vi "Generate stitch tier template.vi"(8 "error in (no error)":errorcluster, 10 "Which tier?":enum16{"Top tier", "Bottom tier"}(ring), 11 "Input image":T1) -> (0 "error out":errorcluster, 3 "Tier image template":T1)   [LabVIEW 2020]
uses:
  <vilib>/vision/Image Controls.llb/IMAQ Image.ctl
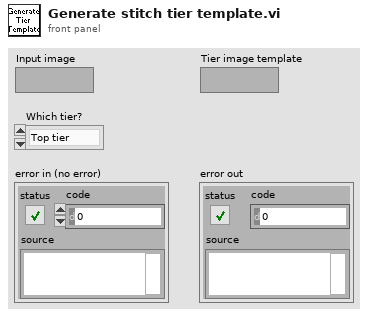
[diagram p1: front panel]
types:
  T1 = typedef "IMAQ Image.ctl" = refnum<image>
  T2 = typedef "Image Type" = u32
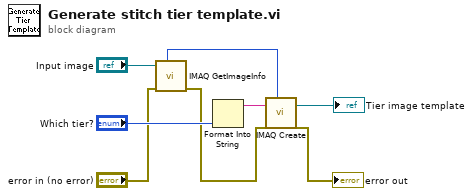
[diagram p0: block diagram]
diagram:
  n1 = call "IMAQ GetImageInfo"("error in (no error)"="error in (no error)", "Image"="Input image") -> ("error out"=w2:errorcluster, "Image Type"=w8:T2)  [unwired: 2 in, 6 out]
  n2 = Format Into String("Which tier?") -> (resulting string=w6:string)  [unwired: 3 in, 1 out]
  n3 = call "IMAQ Create"("Image Name"=w6, "Image Type"=w8, "error in (no error)"=w2) -> ("New Image"=→"Tier image template":T1, "error out"=→"error out":errorcluster)  [unwired: 1 in, 1 out]
